vi "Scripting_SortTerminals.vi"(7 "AbsolutPosition(False)":bool, 11 "Terminals[]":refnum<vi>[](array[refnum])) -> (1 "Ypos":u32[](array[numeric]), 2 "Xpos":u32[](array[numeric]), 3 "TerminalsOut[]":refnum<vi>[](array[refnum]))   [LabVIEW 2014]
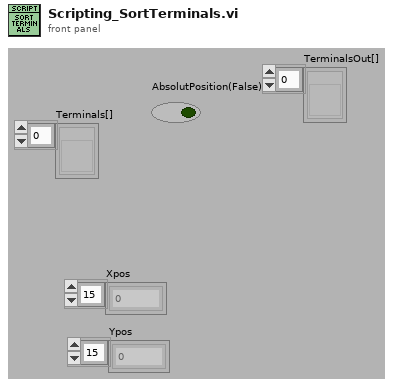
[diagram p1: front panel]
types:
  T1 = typedef "LVPositionTypeDef.ctl" = cluster{"Left":i32, "Top":i32}
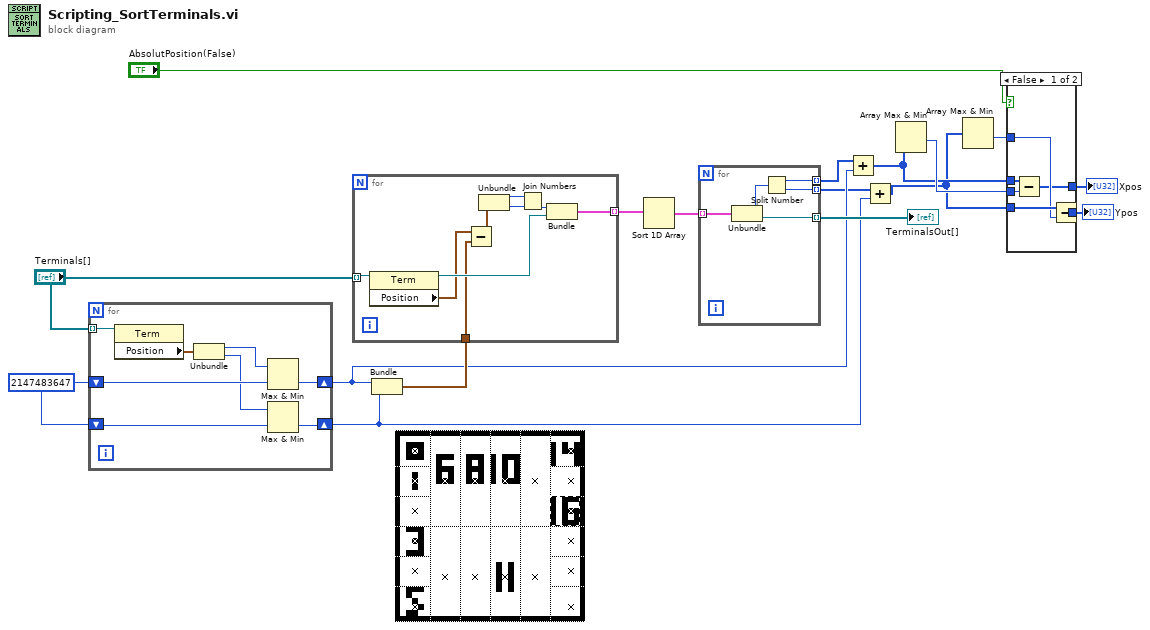
[diagram p0: block diagram]
diagram:
  w8 = 2147483647
  n1 = for {
    tunnel: "Terminals[]" -> [w25] mode=indexing
    shift-right: [w21] -> w6
    shift-left: w8 -> [w22]
    shift-right: [w18] -> w1
    shift-left: w8 -> [w19]
    n2 = property class="Term"(reference=w25) -> ("Position"=w24:T1)  [unwired: 1 in, 2 out]
    n3 = Unbundle(w24) -> ("Left"=w23:i32, "Top"=w20:i32)
    n4 = Max & Min(x=w23, y=w22) -> (min(x,y)=w21:i32)  [unwired: 1 out]
    n5 = Max & Min(x=w20, y=w19) -> (min(x,y)=w18:i32)  [unwired: 1 out]
  }
  n6 = Bundle(w6, w1) -> (w7:cluster{i32, i32})  [unwired: 1 in]
  n7 = for {
    tunnel: "Terminals[]" -> [w34] mode=indexing
    tunnel: [w29] -> w17 mode=indexing
    tunnel: w7 -> [w28]
    n8 = property class="Term"(reference=w34) -> (reference out=w30:refnum<vi>, "Position"=w27:T1)  [unwired: 1 in, 1 out]
    n9 = Subtract(x=w27, y=w28) -> (x-y=w26:T1)
    n10 = Unbundle(w26) -> ("Left"=w33:i32, "Top"=w32:i32)
    n11 = Join Numbers(hi=w33, lo=w32) -> ((hi.lo)=w31:u64)
    n12 = Bundle(w31, w30) -> (w29:cluster{u64, refnum<vi>})  [unwired: 1 in]
  }
  n13 = Sort 1D Array(array=w17) -> (sorted array=w16:cluster{u64, refnum<vi>}[])
  n14 = for {
    tunnel: w16 -> [w39] mode=indexing
    tunnel: [w38] -> w15 mode=indexing
    tunnel: [w36] -> w4 mode=indexing
    tunnel: [w35] -> w3 mode=indexing
    n15 = Unbundle(w39) -> (w37:u64, w38:refnum<vi>)
    n16 = Split Number(x=w37) -> (hi(x)=w36:u32, lo(x)=w35:u32)
  }
  "TerminalsOut[]" <- w15
  n17 = Add(x=w4, y=w6) -> (x+y=w5:u32[])
  n18 = Add(x=w3, y=w1) -> (x+y=w2:u32[])
  n19 = Array Max & Min(array=w5) -> (min value=w14:u32)  [unwired: 3 out]
  n20 = Array Max & Min(array=w2) -> (min value=w13:u32)  [unwired: 3 out]
  n21 = case shown="False" "AbsolutPosition(False)" {
    tunnel: w5 -> [w45 w47]
    tunnel: w14 -> [w44 _]
    tunnel: w2 -> [w43 w46]
    tunnel: w13 -> [w42 _]
    tunnel: [w41 w47] -> w12
    tunnel: [w40 w46] -> w11
    frame False {
      n22 = Subtract(x=w45, y=w44) -> (x-y=w41:u32[])
      n23 = Subtract(x=w43, y=w42) -> (x-y=w40:u32[])
    }
    frame True {
    }
  }
  "Xpos" <- w12
  "Ypos" <- w11
